vi "Send Process Filled Buffer.vi"(7 "Message Priority (Normal)":T2=enum."Normal", 8 "error in (no error)":errorcluster, 10 "Filled Buffers":T1, 11 "Message Enqueuer":refnum<class "Message Enqueuer.lvclass">) -> (0 "error out":errorcluster, 3 "Message Enqueuer out":refnum<class "Message Enqueuer.lvclass">)   [LabVIEW 2020, in "DAQ Interface.lvlib" / "Process Filled Buffer Msg.lvclass"]
doc: "This VI sends the message to an actor."
uses:
  Process Filled Buffer Msg.lvclass
  <vilib>/ActorFramework/Message Enqueuer/Message Enqueuer.lvclass
  <vilib>/ActorFramework/Message Enqueuer/Message Priority.ctl
  TDMS DAQ/TDMS DAQ/Filled Buffers.ctl
  <vilib>/Natan Biesmans/G2CPU GPU and CPU HPC Toolkit/G2CPU Libraries/Async IO/DMA Manager/DMA Manager.lvclass
  C:/Program Files/National Instruments/LabVIEW 2025/vi.lib/ActorFramework/Message/Message.lvclass
  Process Filled Buffer Msg.lvclass/Process Filled Buffer Msg.ctl
  <vilib>/ActorFramework/Message Enqueuer/Message Enqueuer.lvclass/Message Enqueuer.ctl
  <vilib>/ActorFramework/Message Priority Queue/Priority Enqueue.vi
  DAQ Interface/DAQ Interface.lvclass
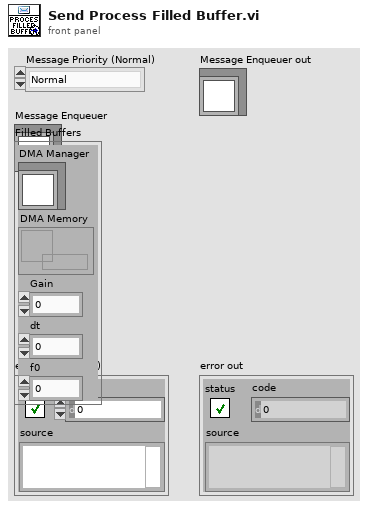
[diagram p1: front panel]
types:
  T1 = typedef "DAQ Interface.lvlib/DAQ Interface.lvclass/Filled Buffers.ctl" = cluster{"DMA Manager":refnum<class "DMA Manager.lvclass">, "DMA Memory":refnum<data-value>, "Gain":dbl, "dt":dbl, "f0":dbl}
  T2 = typedef "Actor Framework.lvlib/Message Enqueuer.lvclass/Message Priority.ctl" = enum16{"Low", "Normal", "High"}
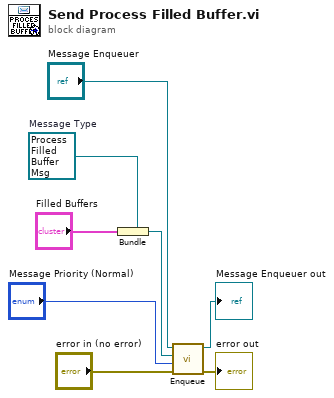
[diagram p0: block diagram]
diagram:
  w5 = refnum<class "Process Filled Buffer Msg.lvclass"> refnum  # Message Type
  n1 = Bundle(cluster=w5, "Filled Buffers") -> (w4:refnum<class "Process Filled Buffer Msg.lvclass">)
  n2 = call <vilib>:"Enqueue.vi"("error in (no error)"="error in (no error)", "Message Priority (Normal)"="Message Priority (Normal)", "Message"=w4, "Message Enqueuer in"="Message Enqueuer") -> ("error out"=→"error out":errorcluster, "Message Enqueuer out"=→"Message Enqueuer out":refnum<class "Message Enqueuer.lvclass">)  [unwired: 6 in]
